vi "Launch Nested.vi"(8 "error in (no error)":errorcluster, 11 "Root Actor in":refnum<class "Root Actor.lvclass">) -> (0 "error out":errorcluster, 3 "Root Actor out":refnum<class "Root Actor.lvclass">)   [LabVIEW 2020, in "Nested Actor.lvlib" / "Root Actor.lvclass"]
uses:
  Root Actor.lvclass
  C:/Program Files (x86)/National Instruments/LabVIEW 2020/vi.lib/ActorFramework/Actor/Actor.lvclass
  Nested Actor/Nested Actor.lvclass
  Root Actor Messages/Rcv  Nested Content Msg/Rcv  Nested Content Msg.lvclass
  E:/NI I Program/Actor Intr Demo/Nested Actor/Nested Actor Messages/Tx Root Content Msg/Tx Root Content Msg.lvclass
  Nested Actor/Nested Actor.lvclass/Nested Actor.ctl
  Root Actor.lvclass/Root Actor.ctl
  <vilib>/ActorFramework/Actor/Actor.lvclass
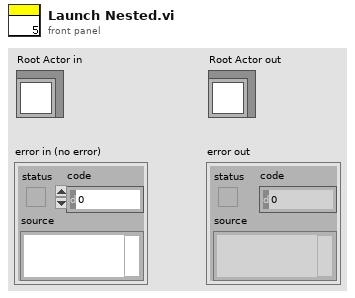
[diagram p1: front panel]
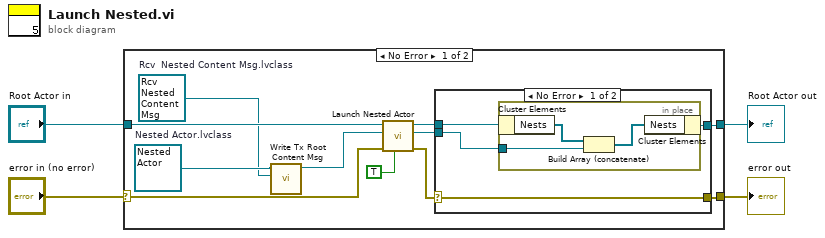
[diagram p0: block diagram]
diagram:
  n1 = case shown="No Error" "error in (no error)" {
    selector: "error in (no error)" -> [w13 w26]
    tunnel: [w8 w26] -> w3
    tunnel: [w11 w25] -> w1
    tunnel: "Root Actor in" -> [w15 w25]
    frame No Error {
      w5 = refnum<class "Rcv  Nested Content Msg.lvclass"> refnum  # Rcv  Nested Content Msg.lvclass
      w7 = refnum<class "Nested Actor.lvclass"> refnum  # Nested Actor.lvclass
      n2 = call "Write Tx Root Content Msg.vi"("Nested Actor.lvlib:Tx Root Content Msg.lvclass"=w5, "Nested Actor in"=w7) -> ("Nested Actor out"=w6:refnum<class "Nested Actor.lvclass">)  [unwired: 9 in]
      n3 = call <vilib>:"Launch Nested Actor.vi"("Open Actor Core front panel? (F)"=TRUE, "error in (no error)"=w13, "Nested Actor"=w6, "Caller Actor in"=w15) -> ("error out"=w9:errorcluster, "Nested Actor's Enqueuer"=w10:refnum<class "Message Enqueuer.lvclass">, "Caller Actor out"=w12:refnum<class "Root Actor.lvclass">)  [unwired: 5 in]
      n4 = case shown="No Error" w9 {
        selector: w9 -> [w16 w24]
        tunnel: w12 -> [w19 w23]
        tunnel: [w18 w23] -> w11
        tunnel: w10 -> [w17 _]
        tunnel: [w16 w24] -> w8
        frame No Error {
          n5 = in-place {
            in-place-border: w17 -> [w20]
            n6 = in-place-cluster #1(w19) -> ("Nests"=w22:refnum<class "Message Enqueuer.lvclass">[])
            n7 = Build Array (concatenate)(w22, w20) -> (w21:refnum<class "Message Enqueuer.lvclass">[])
            n8 = in-place-cluster #1("Nests"=w21) -> (w18:refnum<class "Root Actor.lvclass">)
          }
        }
        frame Error {
        }
      }
    }
    frame Error {
    }
  }
  "error out" <- w3
  "Root Actor out" <- w1
